vi "getDevice.vi"(8 "error in (no error)":errorcluster, 10 "index":i32, 11 "DeviceArray.lvclass in":refnum<class "DeviceArray.lvclass">) -> (0 "error out":errorcluster, 2 "device.lvclass":refnum<class "device.lvclass">, 3 "DeviceArray.lvclass out":refnum<class "DeviceArray.lvclass">)   [LabVIEW 2009, in "Tools.lvlib" / "DatabaseHelpers.lvlib" / "DeviceArray.lvclass"]
uses:
  DeviceArray.lvclass
  device/device.lvclass
  DeviceArray.lvclass/DeviceArray.ctl
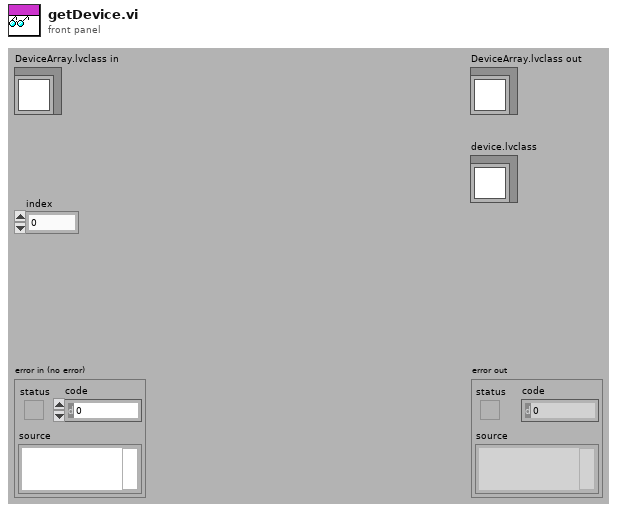
[diagram p1: front panel]
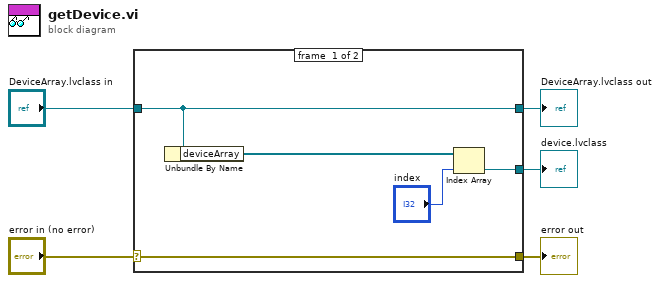
[diagram p0: block diagram]
diagram:
  n1 = case shown="No Error" "error in (no error)" {
    selector: "error in (no error)" -> [w10 w11]
    tunnel: [w10 w11] -> w4
    tunnel: [w9 w12] -> w2
    tunnel: "DeviceArray.lvclass in" -> [w9 w12]
    tunnel: [w6 _] -> w1
    frame #0 {
      n2 = Unbundle By Name(w9) -> ("deviceArray"=w8:refnum<class "device.lvclass">[])
      n3 = Index Array(array=w8, index="index") -> (element=w6:refnum<class "device.lvclass">)
    }
    frame #1 {
    }
  }
  "error out" <- w4
  "DeviceArray.lvclass out" <- w2
  "device.lvclass" <- w1
